vi "DRAFT6.vi"() -> ()   [LabVIEW 2021]
uses:
  5bcb7608-1baa-48ff-8470-29389a5bbc46.vi
  <vilib>/Analysis/3filter.llb/Butterworth Filter (DBL).vi
  <vilib>/Analysis/NI_AALBase.lvlib
  <vilib>/ptbypt/NI_PtbyPt.lvlib
panel:
  out "Waveform Graph 8":dynamicdata(graph)
  out "Waveform Graph 7":dynamicdata(graph)
  out "Array Size 2":u32
  out "Array Size":u32
  out "Elapsed time in ms":u32
  in  "stop":bool
  in  "error in (no error)":errorcluster
  out "error out":errorcluster
  in  "loop 1":i32
  out "Waveform Graph 6":dynamicdata(graph)
  out "Waveform Graph 5":dynamicdata(graph)
  out "Waveform Graph 4":dynamicdata(graph)
  out "Waveform Graph 3":dbl[](graph)
  out "Waveform Graph 2":dynamicdata(graph)
  in  "Boolean":bool
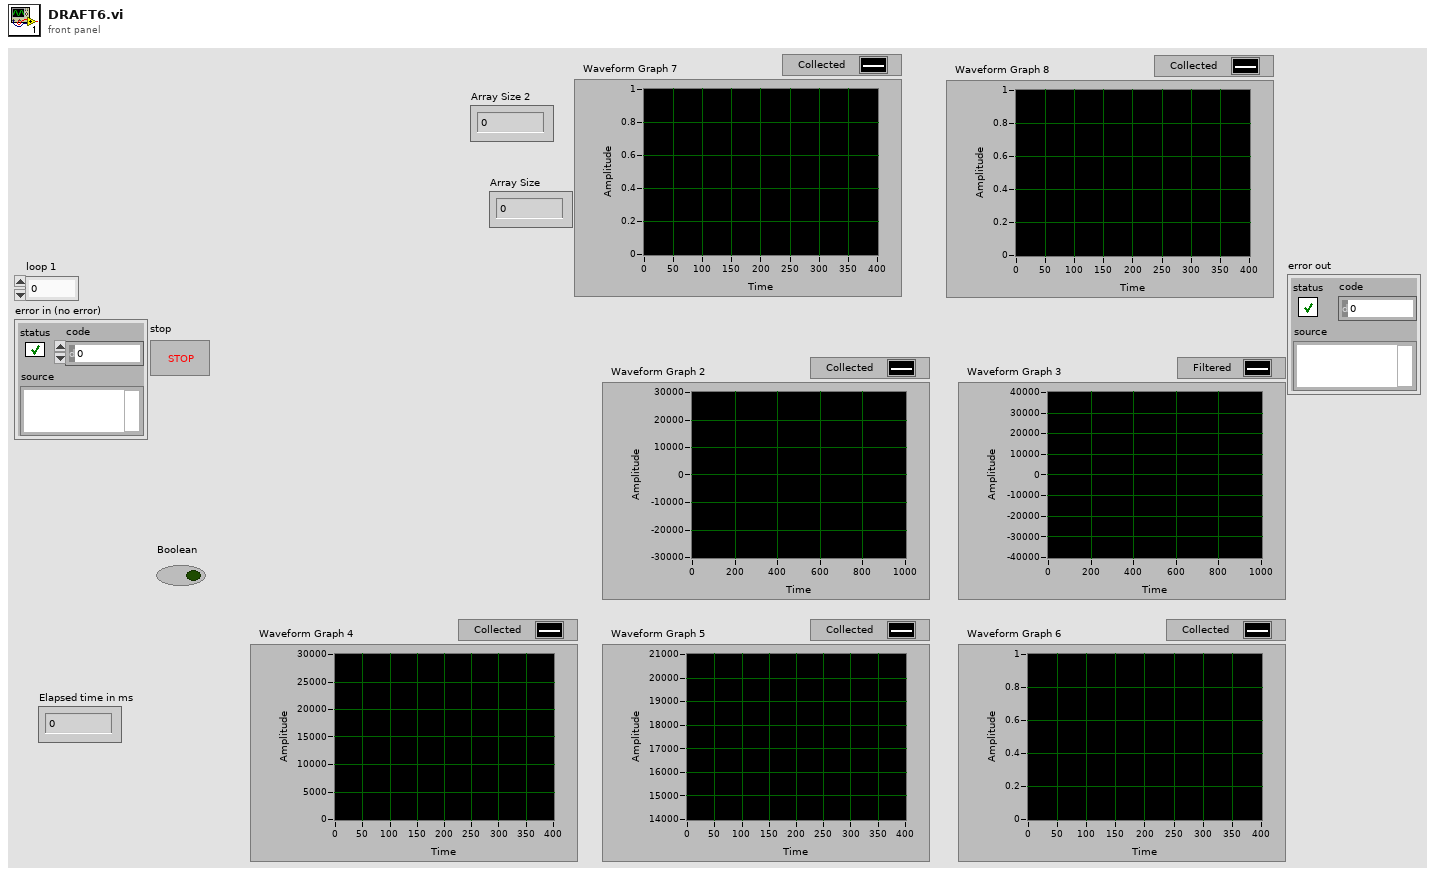
[diagram p1: front panel]
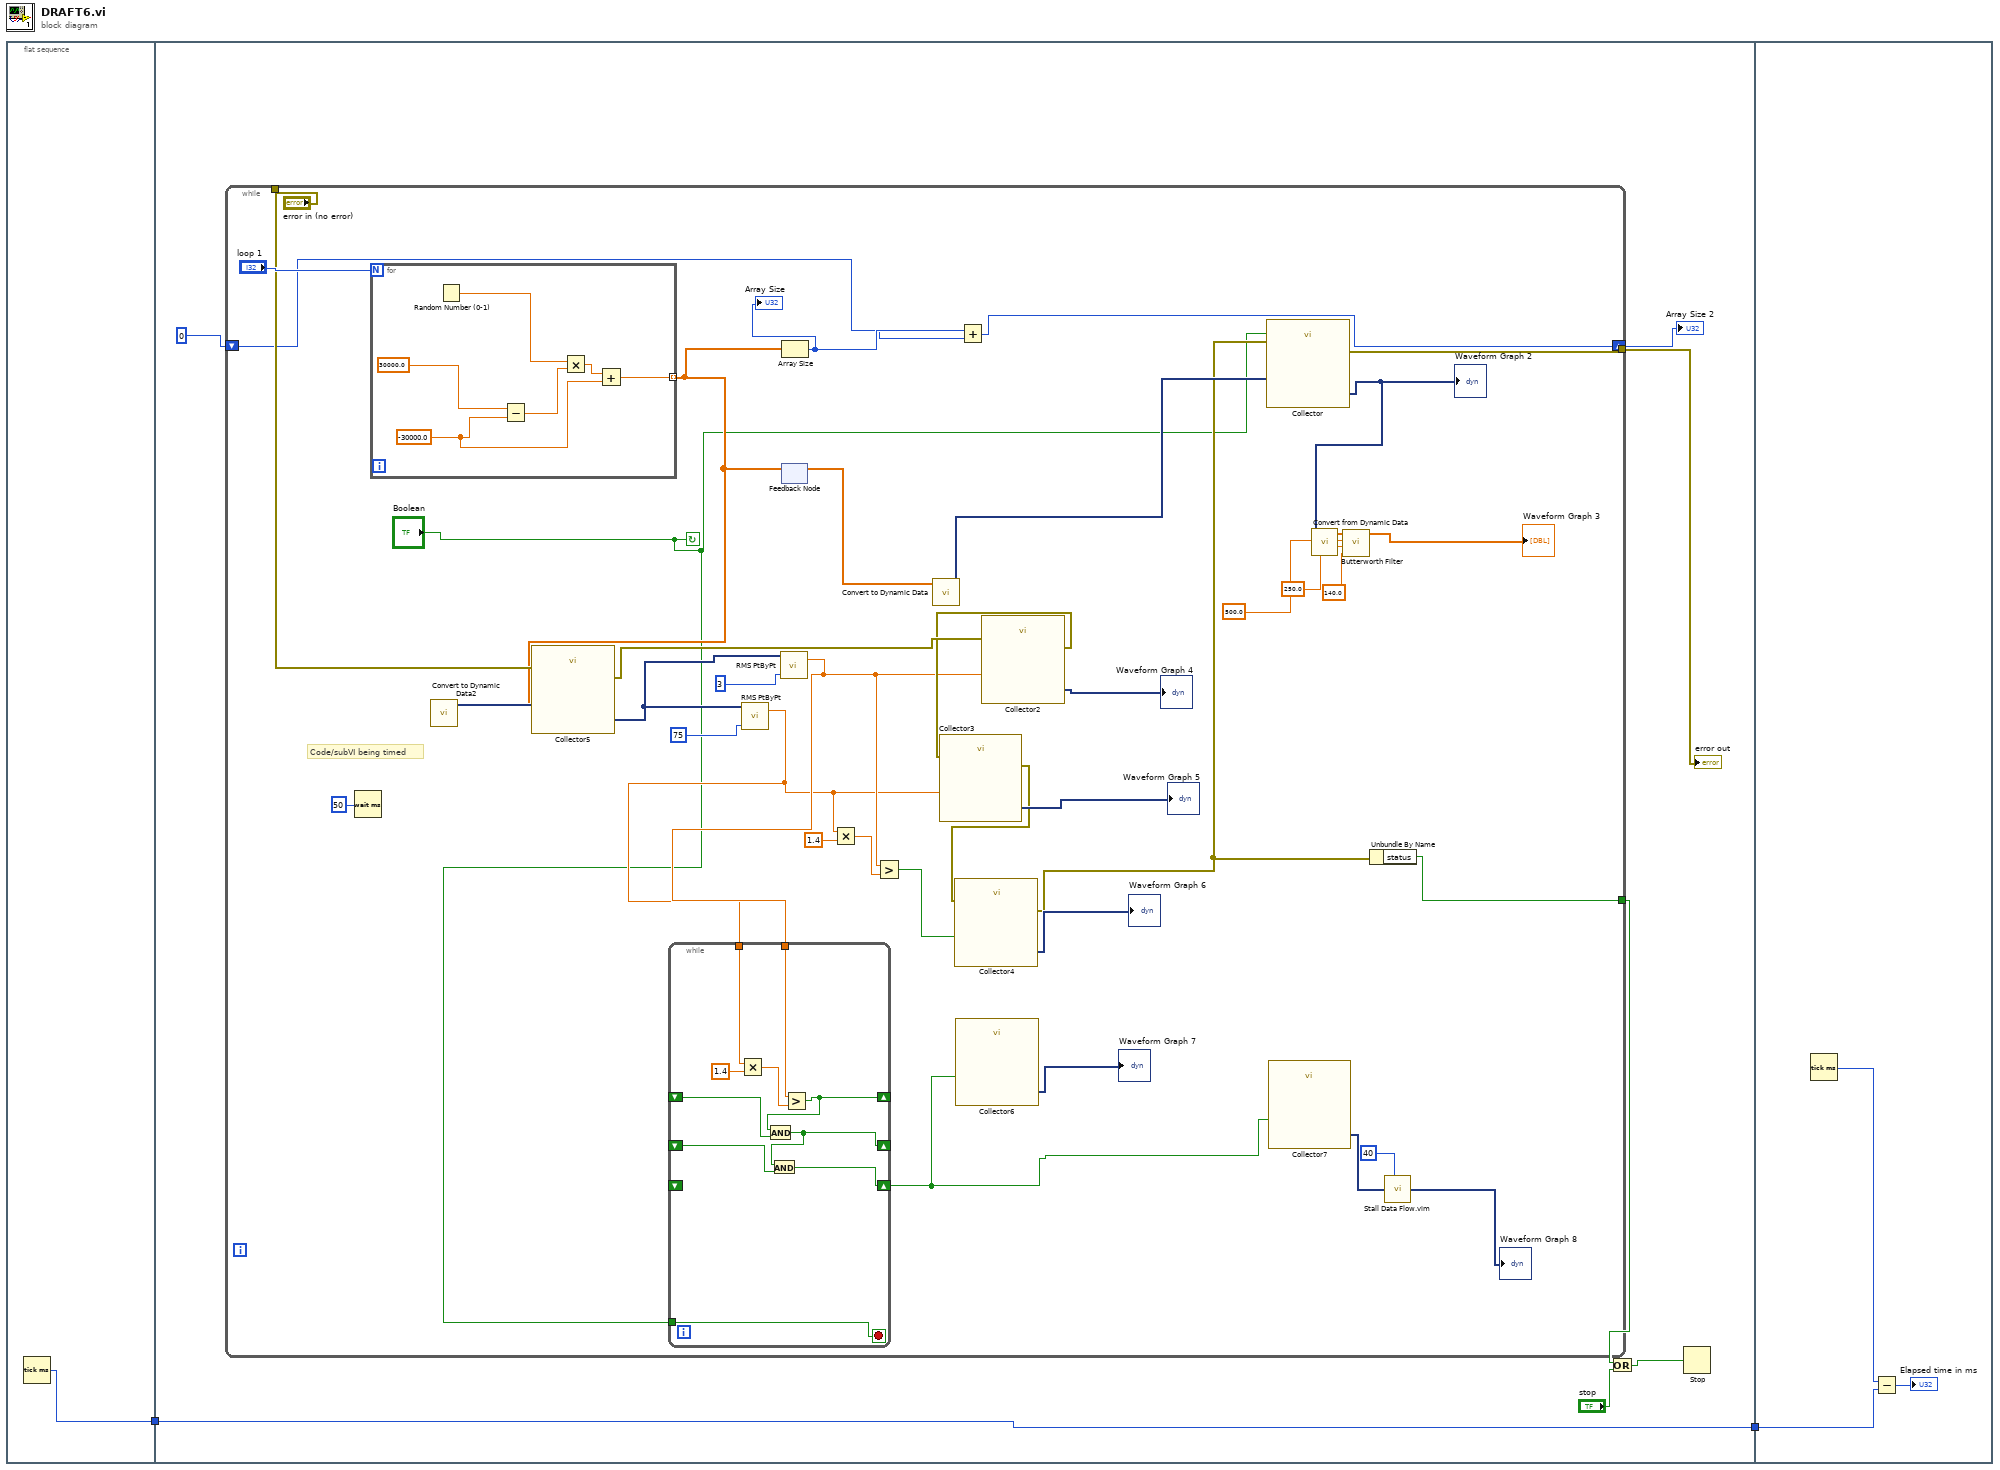
[diagram p0: block diagram]
diagram:
  n1 = flat-sequence {
    tunnel: [w3] -> w2
    tunnel: [w12] -> w1
    tunnel: w2 -> [w12]
    tunnel: w1 -> [w67]
    frame #0 {
      n2 = Tick Count (ms)() -> (millisecond timer value=w3:u32)
    }
    frame #1 {
      # "Code/subVI being timed"
      n3 = while {
        tunnel: "error in (no error)" -> [w32]
        tunnel: [w28] -> w9
        tunnel: [w26] -> w8
        shift-right: [w21] -> w4
        shift-left: 0 -> [w22]
        stop <- "Boolean" continue-if-true
        n4 = for {
          N: "loop 1" -> [_]
          tunnel: [w61] -> w24 mode=indexing
          w63 = -30000.0 ("y")
          n5 = Random Number (0-1)() -> (number: 0 to 1=w62:dbl)
          n6 = Subtract(x=30000.0, y=w63) -> (x-y=w66:dbl)
          n7 = Multiply(x=w62, y=w66) -> (x*y=w65:dbl)
          n8 = Add(x=w65, y=w63) -> (x+y=w61:dbl)
        }
        n9 = call "Convert to Dynamic Data2"("Array"=w24) -> ("Dynamic Data Type"=w34:dynamicdata)  [unwired: 3 in]
        n10 = call "Collector5"("error in (no error)"=w32, "Signals"=w34) -> ("error out"=w31:errorcluster, "Collected Signals"=w33:dynamicdata)  [unwired: 8 in]
        n11 = call <vilib>:"RMS PtByPt.vi"("sample length"=75, "x"=w33) -> ("rms value"=w18:dbl)  [unwired: 2 in, 1 out]
        n12 = call <vilib>:"RMS PtByPt.vi"("sample length"=3, "x"=w33) -> ("rms value"=w19:dbl)  [unwired: 2 in, 1 out]
        n13 = while {
          tunnel: w19 -> [w58]
          tunnel: w18 -> [w57]
          shift-right: [w52] -> _
          shift-left: _ -> [w53]
          shift-right: [w55] -> _
          shift-left: _ -> [w54]
          tunnel: "Boolean" -> [w56]
          shift-right: [w51] -> w16
          shift-left: _ -> [_]
          stop <- w56 stop-if-true
          n14 = Multiply(x=w57, y=1.4) -> (x*y=w59:dbl)
          n15 = Greater?(x=w58, y=w59) -> (0:w55:bool)
          n16 = And(x=w55, y=w54) -> (x .and. y?=w52:bool)
          n17 = And(x=w52, y=w53) -> (x .and. y?=w51:bool)
        }
        n18 = feedback-in #1(w24) -> ()
        n19 = feedback #1() -> (w25:dbl[])  [unwired: 1 in]
        n20 = Array Size(array=w24) -> (size(s)=w23:i32)
        "Array Size" <- w23
        n21 = Multiply(x=w18, y=1.4) -> (x*y=w38:dbl)
        n22 = Greater?(x=w19, y=w38) -> (0:w37:bool)
        n23 = call "Convert to Dynamic Data"("Array"=w25) -> ("Dynamic Data Type"=w42:dynamicdata)  [unwired: 3 in]
        n24 = call "Collector6"("Signals"=w16) -> ("Collected Signals"=→"Waveform Graph 7":dynamicdata)  [unwired: 9 in, 1 out]
        n25 = Add(x=w23, y=w22) -> (x+y=w21:i32)
        n26 = call "Collector2"("error in (no error)"=w31, "Signals"=w19) -> ("error out"=w30:errorcluster, "Collected Signals"=→"Waveform Graph 4":dynamicdata)  [unwired: 8 in]
        n27 = call "Collector3"("error in (no error)"=w30, "Signals"=w18) -> ("error out"=w29:errorcluster, "Collected Signals"=→"Waveform Graph 5":dynamicdata)  [unwired: 8 in]
        n28 = call "Collector4"("error in (no error)"=w29, "Signals"=w37) -> ("error out"=w27:errorcluster, "Collected Signals"=→"Waveform Graph 6":dynamicdata)  [unwired: 8 in]
        n29 = call "Collector"("error in (no error)"=w27, "Enable"="Boolean", "Signals"=w42) -> ("error out"=w28:errorcluster, "Collected Signals"=w45:dynamicdata)  [unwired: 7 in]
        "Waveform Graph 2" <- w45
        n30 = call "Collector7"("Signals"=w16) -> ("Collected Signals"=w15:dynamicdata)  [unwired: 9 in, 1 out]
        n31 = call "Convert from Dynamic Data"("Dynamic Data Type"=w45) -> ("Array"=w47:dbl[])  [unwired: 3 in]
        n32 = call-poly <vilib>:"Butterworth Filter.vi"("low cutoff freq: fl"=140.0, "high cutoff freq: fh"=250.0, "sampling freq: fs"=500.0, "X"=w47) -> ("Filtered X"=→"Waveform Graph 3":dbl[])  [unwired: 4 in, 1 out]
        n33 = Unbundle By Name(w27) -> ("status"=w26:bool)
        n34 = call "Stall Data Flow.vim"("value in"=w15, "milliseconds to wait"=u32 40) -> ("value out"=→"Waveform Graph 8":dynamicdata)  [unwired: 1 out]
      }
      "error out" <- w9
      "Array Size 2" <- w4
      n35 = Wait (ms)(milliseconds to wait=u32 50) -> ()  [unwired: 1 out]
      n36 = Or(x=w8, y="stop") -> (x .or. y?=w6:bool)
      n37 = Stop(stop? (T)=w6) -> ()
    }
    frame #2 {
      n38 = Tick Count (ms)() -> (millisecond timer value=w69:u32)
      n39 = Subtract(x=w69, y=w67) -> (x-y=→"Elapsed time in ms":u32)
    }
  }
